vi "parser.vi"(1 "input":string) -> (7 "temp":string, 9 "vochtigheid":string, 10 "error":bool)   [LabVIEW 2013]
uses:
  <vilib>/regexp/Match Regular Expression.xnode
panel:
  out "read buffer":string
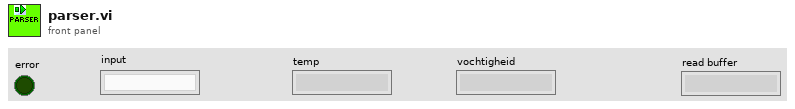
[diagram p1: front panel]
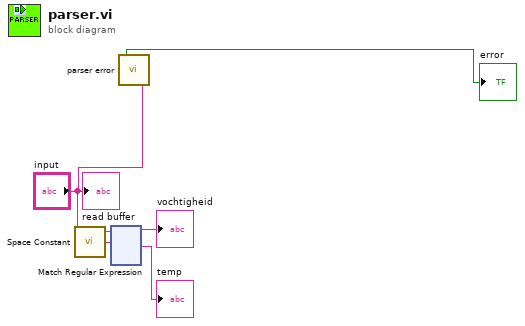
[diagram p0: block diagram]
diagram:
  n1 = call <vilib>:"Space Constant.vi"() -> ("String"=w5:string)
  n2 = xnode "Match Regular Expression"("input string"="input", "regular expression"=w5) -> ("before match"=→"vochtigheid":string, "after match"=→"temp":string)  [unwired: 4 in, 3 out]
  n3 = call "parser error.vi"("string in"="input") -> ("Boolean"=→"error":bool)
  "read buffer" <- "input"
